vi "Pre Launch Init.vi"(11 "Preparation in":refnum<class "Preparation.lvclass">) -> (0 "error out":errorcluster, 3 "Preparation out":refnum<class "Preparation.lvclass">)   [LabVIEW 2015, in "AMS UI.lvlib" / "Preparation.lvclass"]
doc: "(<B>Filename</B>: Actor Framework.lvlib:Actor.lvclass:Pre Launch Init.vi)\n\nDefines behavior that occurs after the Launch Actor method is invoked but before the actor's Actor Core method begins running.\n\nThe Pre Launch Init method is guaranteed to finish before the Launch Actor method returns to its caller and before the actor itself receives any messages. Any references that the Pre Launch Init method obtains are guaranteed to have the same lifetime as the actor itself. Any errors that the Pre Launch Init method returns will abort the launch.\n\nBy default, this method does nothing. A descendant class may override it to define behavior."
uses:
  Preparation.lvclass
  Controls/Register For Notifications Enumerator.ctl
  Preparation.lvclass/Preparation.ctl
  AMS Gas Actor/AMS Gas Actor.lvclass
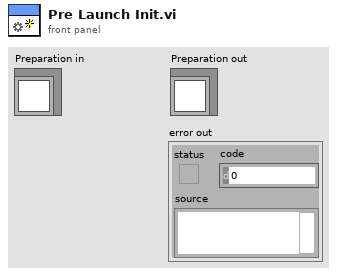
[diagram p1: front panel]
types:
  T1 = typedef "Register For Notifications Enumerator.ctl" = enum16{"Storage Tubes", "Storage Valves", "Sample Lines", "Syringe Container", "Capillary Container", "Preparation Line"}
  T2 = typedef "Sample Container.ctl" = cluster{"Sample In":refnum<k21>, "Sample Name":refnum<k21>, "Ti Cathode":refnum<k21>, "SampleQ":refnum<queue>}
  T3 = typedef "FP Control Refs Cluster.ctl" = cluster{"Liquid N Valve References":T4, "Main Line Valve Refs":T5, "Transfer Line Container":refnum<vi>, "Storage Containers":refnum<vi>[], "Sample Refs":T6, "Syringe Ctrl Refs ":T7, "Baratrons Chart":refnum<vi>, "Capillary Container":refnum<vi>, "Preparation Container":refnum<vi>, "Monkey Mode":refnum<vi>}
  T4 = typedef "Liquid N Valve Ref Cluster.ctl" = cluster{"Cold Bath H2O HV 100":refnum<vi>, "Cold Bath Cleaning HV 101":refnum<vi>, "Cold Bath Storage 1 HV 102":refnum<vi>, "Cold Bath Storage 2 HV 103":refnum<vi>, "Cold Bath Storage 3 HV 104":refnum<vi>, "Cold Bath Storage 4 HV 105":refnum<vi>, "Cold Bath Syringe HV 106":refnum<vi>, "Liquid N Master Valve HV 107":refnum<vi>}
  T5 = typedef "Main Line Valve Ref Cluster.ctl" = cluster{"Turbo Valve DV313":refnum<vi>, "Prep Line Valve 0 DV300":refnum<vi>, "Storage Valves":refnum<vi>[]}
  T6 = typedef "Sample Valve Refs.ctl" = cluster{"Valves":cluster{"Sample 5 DV318":refnum<vi>, "Sample 4 DV317":refnum<vi>, "Sample 3 DV316":refnum<vi>, "Sample 2 DV315":refnum<vi>, "Sample 1 DV314":refnum<vi>}, "Lines":cluster{"Sample 1":refnum<vi>, "Sample 2":refnum<vi>, "Sample 3":refnum<vi>, "Sample 4":refnum<vi>, "Sample 5":refnum<vi>}}
  T7 = typedef "Syringe Ctrl Refs.ctl" = cluster{"Syringe Home":refnum<vi>, "Syringe Freeze":refnum<vi>, "Syringe TC":refnum<vi>, "Syringe Container":refnum<vi>}
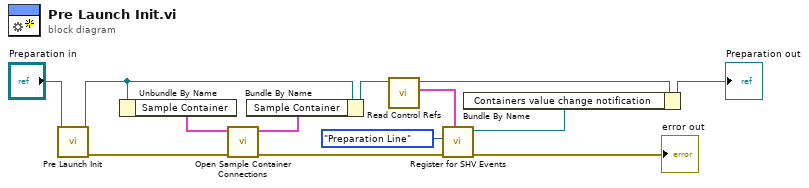
[diagram p0: block diagram]
diagram:
  n1 = call-parent "Pre Launch Init.vi"("eActor in"="Preparation in") -> ("error out"=w7:errorcluster, "eActor out"=w5:refnum<class "Preparation.lvclass">)  [unwired: 9 in]
  n2 = Unbundle By Name(w5) -> ("Sample Container"=w8:T2)
  n3 = call "Open Sample Container Connections.vi"("error in (no error)"=w7, "Container in"=w8) -> ("error out"=w10:errorcluster, "Container out"=w9:T2)  [unwired: 8 in]
  n4 = Bundle By Name(cluster=w5, "Sample Container"=w9) -> (w4:refnum<class "Preparation.lvclass">)
  n5 = call-dynamic "Read Control Refs.vi"("AMS Gas Actor in"=w4) -> ("Control Refs"=w13:T3, "AMS Gas Actor out"=w3:refnum<class "Preparation.lvclass">)  [unwired: 9 in]
  n6 = call "Register for SHV Events.vi"("Control Refs"=w13, "error in (no error)"=w10, "Register for"=Register_For_Notifications_Enumerator."Preparation Line") -> ("error out"=→"error out":errorcluster, "Containers SHV change notification"=w11:refnum<user-event>)  [unwired: 7 in]
  n7 = Bundle By Name(cluster=w3, "Containers value change notification"=w11) -> (→"Preparation out":refnum<class "Preparation.lvclass">)
